vi "Correct_Position.vi"(8 "error in (no error)":errorcluster, 10 "Car Position Slider":u8, 11 "Enum":T1) -> (0 "error out":errorcluster, 3 "In Correct Position?":bool)   [LabVIEW 2021]
doc: "VI determines if the car is in the correct position for the wash step"
uses:
  Controls/states.ctl
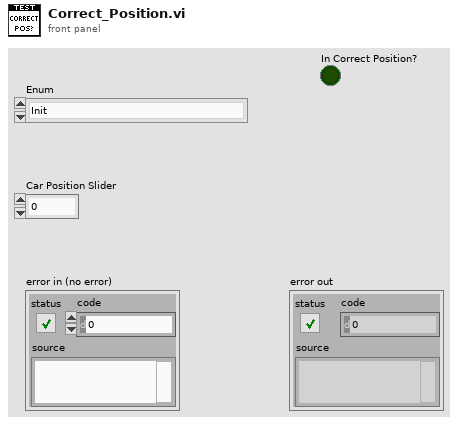
[diagram p1: front panel]
types:
  T1 = typedef "states.ctl" = enum16{"Init", "Select Wash Options", "Configure Options", "Under Body Wash", "Bug Remover", "Pre-Soak", "High Pressure Wash", "Low Pressure Wax", "Spot Free Rinse", "Tire Shine Foam", "Air Dry", "Skip", "Exit", "Stop"}
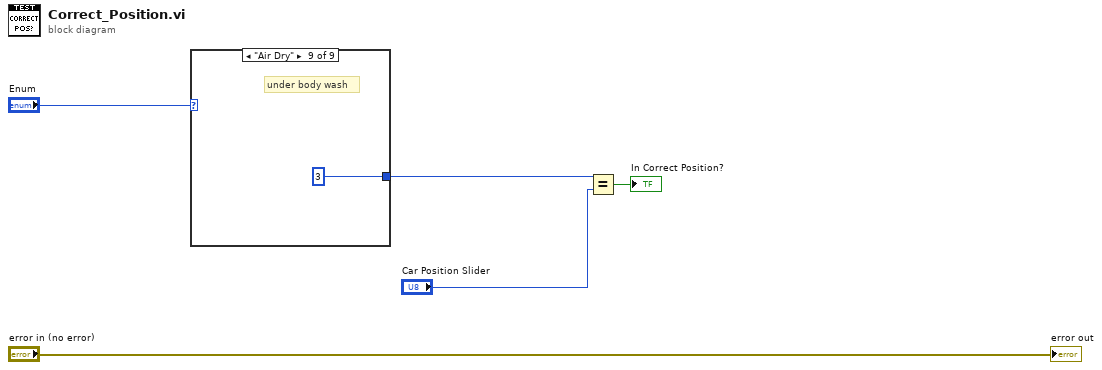
[diagram p0: block diagram]
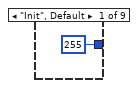
[diagram p2: hidden frame]
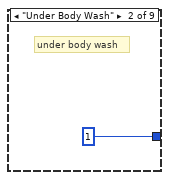
[diagram p3: hidden frame]
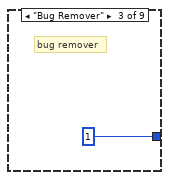
[diagram p4: hidden frame]
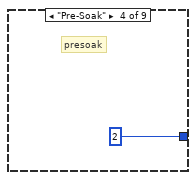
[diagram p5: hidden frame]
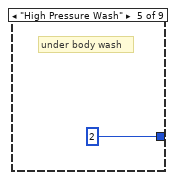
[diagram p6: hidden frame]
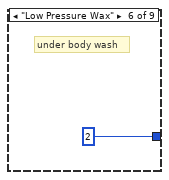
[diagram p7: hidden frame]
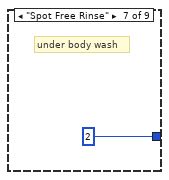
[diagram p8: hidden frame]
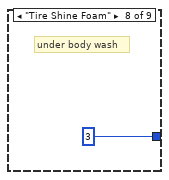
[diagram p9: hidden frame]
diagram:
  n1 = case shown="\"Air Dry\"" "Enum" {
    tunnel: [u8 255 ("x") u8 1 ("x") u8 1 ("x") u8 2 ("x") u8 2 ("x") u8 2 ("x") u8 2 ("x") u8 3 ("x") u8 3 ("x")] -> w2
    frame "Init", Default {
    }
    frame "Under Body Wash" {
      # "under body wash"
    }
    frame "Bug Remover" {
      # "bug remover"
    }
    frame "Pre-Soak" {
      # "presoak"
    }
    frame "High Pressure Wash" {
      # "under body wash"
    }
    frame "Low Pressure Wax" {
      # "under body wash"
    }
    frame "Spot Free Rinse" {
      # "under body wash"
    }
    frame "Tire Shine Foam" {
      # "under body wash"
    }
    frame "Air Dry" {
      # "under body wash"
    }
  }
  n2 = Equal?(x=w2, y="Car Position Slider") -> (x = y?=→"In Correct Position?":bool)
  "error out" <- "error in (no error)"
